vi "Imaq_fgv.vi"(7 "cmd":enum16{"create", "close", "read"}(ring), 8 "error in":errorcluster) -> (0 "error out":errorcluster caption="error our", 3 "New Image":T1)   [LabVIEW 2016]
uses:
  <vilib>/vision/Image Controls.llb/IMAQ Image.ctl
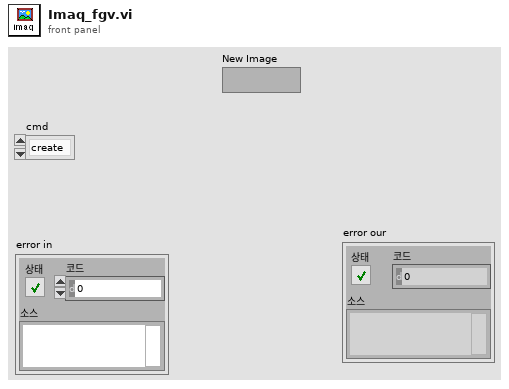
[diagram p1: front panel]
types:
  T1 = typedef "IMAQ Image.ctl" = refnum<image>
  T2 = typedef "Image Type" = u32
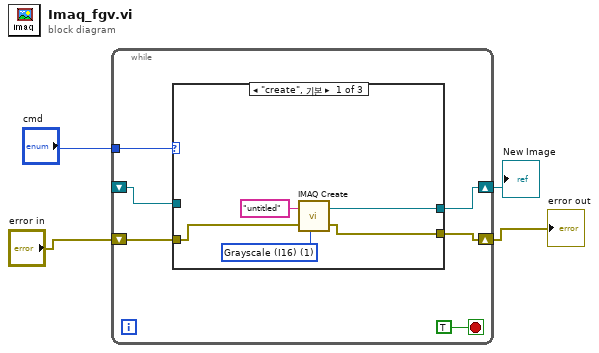
[diagram p0: block diagram]
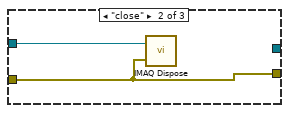
[diagram p2: hidden frame]
diagram:
  n1 = while {
    tunnel: "cmd" -> [w9]
    shift-right: [w8] -> w2
    shift-left: "error in" -> [w7]
    shift-right: [w5] -> w1
    shift-left: _ -> [w6]
    stop <- TRUE stop-if-true
    n2 = case shown="\"create\", 기본" w9 {
      tunnel: [w14 w17 w19] -> w8
      tunnel: w7 -> [w15 w17 w19]
      tunnel: w6 -> [_ w16 w18]
      tunnel: [w12 _ w18] -> w5
      frame "create", Default {
        w11 = T2 1 items=["Grayscale (U8)", "Grayscale (I16)", "Grayscale (SGL)", "Complex (CSG)", "RGB (U32)", "HSL (U32)", "RGB (U64)", "Grayscale (U16)"] ("Image Type")
        n3 = call "IMAQ Create"("Image Name"="untitled", "Image Type"=w11, "error in (no error)"=w15) -> ("New Image"=w12:T1, "error out"=w14:errorcluster)  [unwired: 2 in]
      }
      frame "close" {
        n4 = call "IMAQ Dispose"("Image"=w16, "error in (no error)"=w17) -> ()  [unwired: 4 in, 1 out]
      }
      frame "read" {
      }
    }
  }
  "error out" <- w2
  "New Image" <- w1
